vi "ResolveConfig.vi"(8 "error in (no error)":errorcluster, 11 "LogManager in":refnum<class "LogManager.lvclass">) -> (0 "error out":errorcluster, 3 "LogManager out":refnum<class "LogManager.lvclass">)   [LabVIEW 2026, in "Lumberjack.lvlib" / "LogManager.lvclass"]
doc: "Resolve the LogManager's effective configuration on startup: read the stashed launch inputs (initial global threshold, default file appender config, config file path, host application path) and call Resolve (Merge with the JSON file over the baseline, Validate, produce native ResolvedConfig). Store the result as resolvedConfig. A missing config file is a non-fatal warning (baseline stands); a present but unparseable file is fatal. Called once by Actor Core on entry (SRS-LMBR-044-051)."
uses:
  LogManager.lvclass
  LogManager.lvclass/LogManager.ctl
  Lumberjack.lvlib
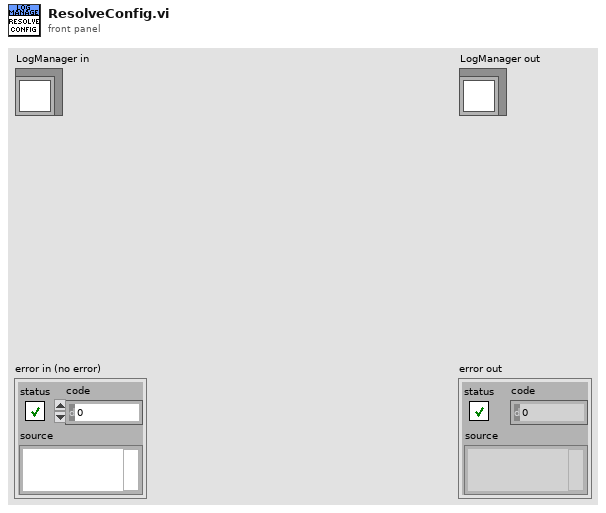
[diagram p1: front panel]
types:
  T1 = typedef "Lumberjack.lvlib/Severity.ctl" = enum16{"OFF", "FATAL", "ERROR", "WARN", "INFO", "DEBUG", "TRACE", "ALL"}
  T2 = typedef "Lumberjack.lvlib/FileAppenderConfig.ctl" = cluster{"common":T3, "file":T7}
  T3 = typedef "Lumberjack.lvlib/AppenderConfig.ctl" = cluster{"id":string, "threshold":T1, "filter":T4, "queueBound":i32, "dropPolicy":T6, "useUTC":bool}
  T4 = typedef "Lumberjack.lvlib/Filter.ctl" = cluster{"mode":T5, "levelMin":T1, "levelMax":T1, "tagPrefix":string}
  T5 = typedef "Lumberjack.lvlib/FilterMode.ctl" = enum16{"Mirror", "Routed"}
  T6 = typedef "Lumberjack.lvlib/DropPolicy.ctl" = enum16{"DropOldest", "DropNewest", "LevelAware"}
  T7 = typedef "Lumberjack.lvlib/FileConfig.ctl" = cluster{"rootFolder":path, "maxFileSize":i64, "maxFileCount":i32, "baseName":string, "extension":string, "delimiter":string, "calendarFolderTree":bool}
  T8 = typedef "Lumberjack.lvlib/LumberjackConfig.ctl" = cluster{"schemaVersion":string, "globalThreshold":T1, "defaultFileAppender":T2}
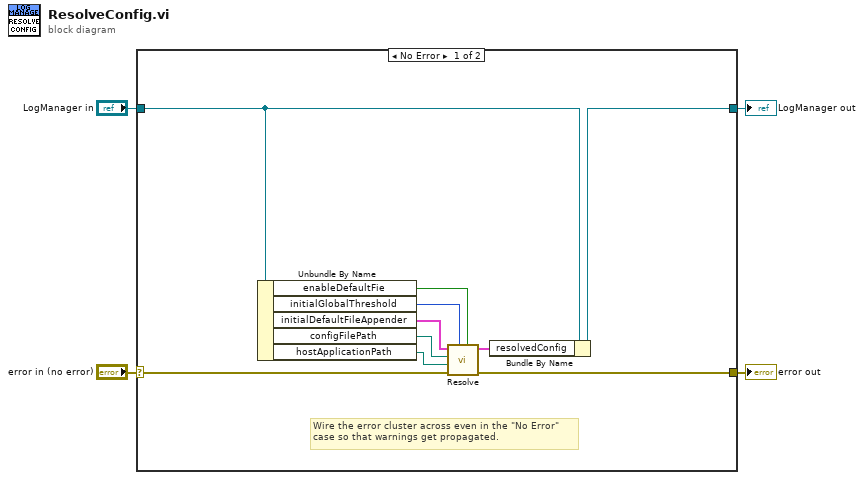
[diagram p0: block diagram]
diagram:
  n1 = case shown="No Error" "error in (no error)" {
    selector: "error in (no error)" -> [w13 w16]
    tunnel: [w12 w16] -> w3
    tunnel: [w6 w15] -> w1
    tunnel: "LogManager in" -> [w8 w15]
    frame No Error {
      # "Wire the error cluster across even in the \"No Error\"\ncase so that warnings get propagated."
      n2 = Unbundle By Name(w8) -> ("enableDefaultFie"=w5:bool, "initialGlobalThreshold"=w14:T1, "initialDefaultFileAppender"=w9:T2, "configFilePath"=w10:path, "hostApplicationPath"=w11:path)
      n3 = call "Resolve.vi"("enableDefaultFile"=w5, "GlobalThreshold"=w14, "error in (no error)"=w13, "HostApplicationPath"=w11, "ConfigFilePath"=w10, "DefaultFileAppenderConfig"=w9) -> ("error out"=w12:errorcluster, "ResolvedConfig"=w7:T8)  [unwired: 4 in]
      n4 = Bundle By Name(cluster=w8, "resolvedConfig"=w7) -> (w6:refnum<class "LogManager.lvclass">)
    }
    frame Error {
    }
  }
  "error out" <- w3
  "LogManager out" <- w1
